vi "Scale Encoder IP to Array Index.vi"(7 "Micropulse # In":i32, 9 "Inspection Point Location":u32, 10 "Scan definition":T1 {"Inspection Resolution" format="%#_6f"; "Scan Start" format="%#_6f"; "Scan Length" format="%#_6f"}, 11 "Axis No.":u8=1 min=1 max=4) -> (1 "Absolute Location":dbl, 3 "B-Scan index":i32)   [LabVIEW 2026, in "MicroPulse_Driver.lvlib"]
uses:
  MicroPulse_Driver.lvlib
  Data/Datatypes/MP - fly scan range.ctl
  Data/Datatypes/MP - inspection direction.ctl
  <instrlib>/Micropulse/Micropulse.lvlib
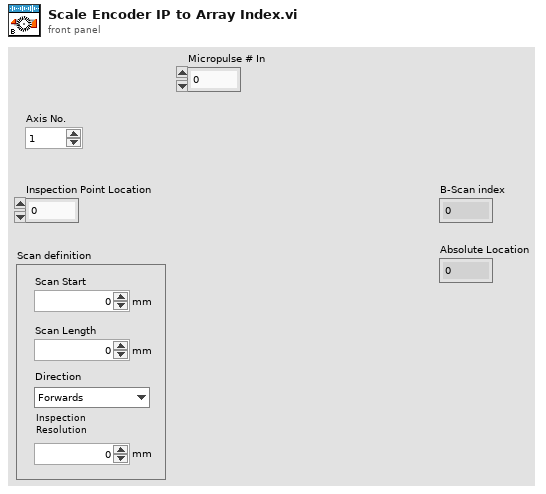
[diagram p1: front panel]
types:
  T1 = typedef "Micropulse.lvlib/MP - fly scan range.ctl" = cluster{"Scan Start":dbl, "Scan Length":dbl, "Inspection Resolution":dbl, "Direction":T2}
  T2 = typedef "Micropulse.lvlib/MP - inspection direction.ctl" = enum16{"Forwards", "Backwards"}
  T3 = typedef "Micropulse.lvlib/MP-Registry Data-Cluster.ctl" = cluster{"Instrument Type":T4, "Serial #":u64, "Sample Frequency":T5, "dt (us)":dbl, "DOF":T6, "Material Velocity":dbl, "Asynch Reads":T7, "NUM of Tests":u32, "System Details":T8, "Gates":T10[], "Encoders":T17[], "CMD LUT":variant, "Command List":string}
  T4 = typedef "Micropulse.lvlib/MP - instrument type.ctl" = enum16{"MicroPulse 5", "LT1", "LT2", "LTPA", "MPLT", "MicroPulse 6", "PipeScanner", "<MicroPulse>", "Micropulse 4", "Simulated Data"}
  T5 = typedef "Micropulse.lvlib/MP - sample frequency.ctl" = enum16{"Use Default", "200MHz (LT2 only)", "100MHz", "50MHz", "25MHz", "10MHz"}
  T6 = typedef "Micropulse.lvlib/MP - data output format.ctl" = enum16{"", "8-bit Mode", "10-bit Mode", "12-bit Mode", "16-bit Mode", "8-bit Log Mode", "12-bit Packed Mode"}
  T7 = typedef "Micropulse.lvlib/MP - asynch read mode.ctl" = enum16{"Disabled", "Enabled"}
  T8 = typedef "Micropulse.lvlib/MP - general system status.ctl" = cluster{"System Type":T4, "Serial No.":u64, "Channels":cluster{"Conv":u8, "PA":u16, "Extra":u32}, "Sample Frequency":cluster{"Default":u8, "Actual":u8}, "Software Versions":string, "Data Output Format":cluster{"Default":T6, "Actual":T6}, "Temperatures":cluster{"System":u8, "Processor":u8, "Slave Sys":u8, "Slave Proc":u8}, "Tx Buffer Size":u32, "System Error":string, "No. of Cards":u8, "DAC Gain":i16, "Uptimes":cluster{"since Power":u32, "since RSTS":u32, "since SRST":u32}, "Voltages":cluster{"Nominal":dbl, "Measured":dbl, "Difference":dbl}[], "Interface Cards":T9[]}
  T9 = typedef "Micropulse.lvlib/MP - interface card status.ctl" = cluster{"Status":u8, "Map":u8, "Board - T":u8, "FPGA - T":u8, "PAIF Status":string, "Version":string}
  T10 = typedef "Micropulse.lvlib/MP - Registry Gates.ctl" = cluster{"Display Gate":T11, "ETM Mode":T12, "Echo Gate":T13, "Insp Gates":T14[]}
  T11 = typedef "Micropulse.lvlib/MP - display gate.ctl" = cluster{"Start":dbl, "Length":dbl}
  T12 = typedef "Micropulse.lvlib/MP - echo gate mode.ctl" = enum16{"Echo Trigger OFF", "Echo Gate Display Mode", "Echo Trigger ON", "Multi Gate or FMC Mode", "Reserved", "PA - Echo Trigger ON"}
  T13 = typedef "Micropulse.lvlib/MP - echo gate parameters.ctl" = cluster{"Start (us)":dbl, "Length (us)":dbl, "Threshold":u16, "Colour":u32}
  T14 = typedef "Micropulse.lvlib/MP - multigate inspection gate parameters.ctl" = cluster{"Start (us)":dbl, "Length (us)":dbl, "Threshold":u16, "Enabled?":bool, "Max # Peaks":u16, "Hysteresis":T15, "Mode":T16, "Inverted?":bool, "Colour ":u32}
  T15 = typedef "Micropulse.lvlib/MP - hysteresis level.ctl" = enum16{"None", "3dB", "6dB", "9dB", "12dB"}
  T16 = typedef "Micropulse.lvlib/MP - multigate mode.ctl" = enum16{"1st Peak in Gate", "Largest Peak In Gate", "All Peaks In Gate", "1st Threshold Crossing"}
  T17 = typedef "Micropulse.lvlib/MP - encoder settings.ctl" = cluster{"Encoder Type":T18, "Counts/mm":u32, "Enable Termination?":bool, "Multiplier":u32, "Backlash Period (s)":dbl, "Encoder Filter":u32}
  T18 = typedef "Micropulse.lvlib/MP - encoder type.ctl" = enum16{"Quadrature", "Step/Direction"}
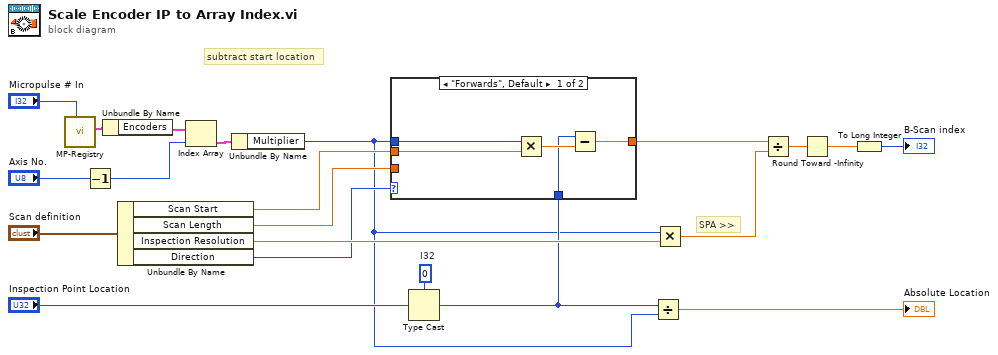
[diagram p0: block diagram]
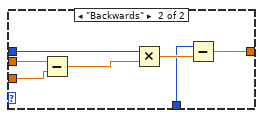
[diagram p2: hidden frame]
diagram:
  w6 = 0  # I32
  # "subtract start location"
  # "SPA >>"
  n1 = call "MP-Registry.vi"("Micropulse # In"="Micropulse # In") -> ("Micropulse Data"=w16:T3)  [unwired: 7 in, 3 out]
  n2 = Decrement(x="Axis No.") -> (x-1=w4:u8)
  n3 = Unbundle By Name(w16) -> ("Encoders"=w15:T17[])
  n4 = Unbundle By Name("Scan definition") -> ("Scan Start"=w12:dbl, "Scan Length"=w7:dbl, "Inspection Resolution"=w21:dbl, "Direction"=w8:T2)
  n5 = Index Array(array=w15, index=w4) -> (element=w14:T17)
  n6 = Unbundle By Name(w14) -> ("Multiplier"=w2:u32)
  n7 = Type Cast(type=w6, x="Inspection Point Location") -> (*(type *) &x=w3:i32)
  n8 = case shown="\"Forwards\", Default" w8 {
    tunnel: w12 -> [w26 w33]
    tunnel: w3 -> [w24 w31]
    tunnel: [w23 w30] -> w10
    tunnel: w2 -> [w22 w29]
    tunnel: w7 -> [_ w27]
    frame "Forwards", Default {
      n9 = Multiply(x=w22, y=w26) -> (x*y=w25:dbl)
      n10 = Subtract(x=w24, y=w25) -> (x-y=w23:dbl)
    }
    frame "Backwards" {
      n11 = Subtract(x=w33, y=w27) -> (x-y=w28:dbl)
      n12 = Multiply(x=w29, y=w28) -> (x*y=w32:dbl)
      n13 = Subtract(x=w31, y=w32) -> (x-y=w30:dbl)
    }
  }
  n14 = Divide(x=w3, y=w2) -> (x/y=→"Absolute Location":dbl)
  n15 = Multiply(x=w2, y=w21) -> (x*y=w13:dbl)
  n16 = Divide(x=w10, y=w13) -> (x/y=w17:dbl)
  n17 = Round Toward -Infinity(1:w17) -> (0:w9:dbl)
  n18 = To Long Integer(number=w9) -> (32bit integer=→"B-Scan index":i32)
